vi "MotionProfileUpdater.vi"(11 "Main MP Controller In":T1={"DeviceStatus"={"status"=FALSE, "code"=0, "source"=""}, "Type"=enum."PWM", "PWM"={"PWM Channel"=enum."Invalid", "DeadBand"={"Name"="", "maxPositivePwm"=0, "minPositivePwm"=0, "centerPwm"=0, "maxNegativePwm"=0, "minNegativePwm"=0, "angularRange"=0}}, "CAN"={"Device Number"=0, "SetOutput VI Ref"=variant(enum8{"Percent VBus", "Current", "Speed", "Position", "Voltage"} enum."Percent VBus"), "GetOutput VI Ref"=variant(refnum<k1> refnum), "Enable VI Ref"=variant(dbl 12.0), "Disable VI Ref"=variant(enum8{"Percent VBus", "Speed", "Position", "Slave", "Unchanged / Invalid", "Voltage Compensation", "Current", "Motion Profile"} enum."Percent VBus"), "Data"=variant}, "Invert"=FALSE, "DIO PWM"={"PWM \"Enable\" Channel"=enum."Invalid", "DIOChannel"=enum."Invalid", "PWM Rate"=0.0}}) -> ()   [LabVIEW 2017]
uses:
  <vilib>/Rock Robotics/WPI/MotorControl/WPI_MotorControlDeviceRef.ctl
  <vilib>/Rock Robotics/WPI/MotorControl/WPI_MotorControlType.ctl
  <vilib>/Rock Robotics/SystemInterfaces/DIO/FPGA_DIOPWMChannel.ctl
  <vilib>/Rock Robotics/WPI/PWM/WPI_PWMDeadband.ctl
  <vilib>/Rock Robotics/SystemInterfaces/DIO/FPGA_DIOChannel.ctl
  TrajectoryPointCluster.ctl
  <vilib>/Rock Robotics/WPI/ThirdParty/Phoenix-LabVIEW/Motor Controller/Controls/CTRE_Phoenix_MotorControl_StatusFrameEnhanced.ctl
  <vilib>/Rock Robotics/WPI/ThirdParty/Phoenix-LabVIEW/Motor Controller/Controls/CTRE_Phoenix_MotorControl_ControlFrameEnhanced.ctl
  <vilib>/Rock Robotics/WPI/ThirdParty/Phoenix-LabVIEW/Motor Controller/Controls/CTRE_Phoenix_MotorControl_TrajectoryPointTimeDur.ctl
  MotionProfileController.vi
  Constants.vi
panel:
  out "Loop Rate (ms)":u32
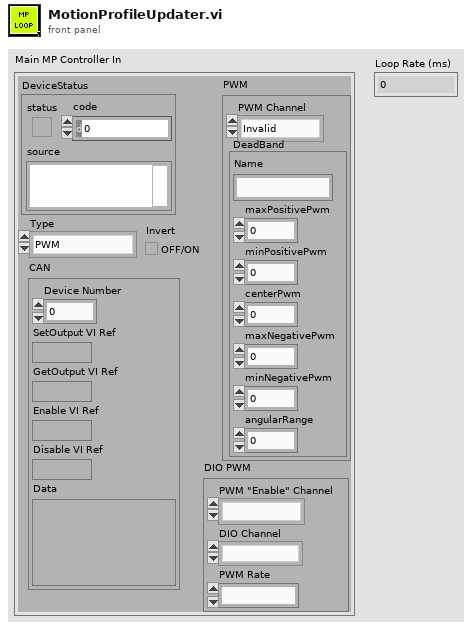
[diagram p1: front panel]
types:
  T1 = typedef "WPI_MotorControlDeviceRef.ctl" = cluster{"DeviceStatus":errorcluster, "Type":T2, "PWM":cluster{"PWM Channel":T3, "DeadBand":T4}, "CAN":cluster{"Device Number":u8, "SetOutput VI Ref":variant, "GetOutput VI Ref":variant, "Enable VI Ref":variant, "Disable VI Ref":variant, "Data":variant}, "Invert":bool, "DIO PWM":cluster{"PWM \"Enable\" Channel":T3, "DIOChannel":T5, "PWM Rate":dbl}}
  T2 = typedef "WPI_MotorControlType.ctl" = enum16{"PWM", "CAN", "DIO PWM"}
  T3 = typedef "FPGA_DIOPWMChannel.ctl" = enum8{"PWM 0", "PWM 1", "PWM 2", "PWM 3", "PWM 4", "PWM 5", "PWM 6", "PWM 7", "PWM 8", "PWM 9", "PWM MXP 0", "PWM MXP 1", "PWM MXP 2", "PWM MXP 3", "PWM MXP 4", "PWM MXP 5", "PWM MXP 6", "PWM MXP 7", "PWM MXP 8", "PWM MXP 9", "Invalid"}
  T4 = typedef "WPI_PWMDeadband.ctl" = cluster{"Name":string, "maxPositivePwm":i32, "minPositivePwm":i32, "centerPwm":i32, "maxNegativePwm":i32, "minNegativePwm":i32, "angularRange":u16}
  T5 = typedef "FPGA_DIOChannel.ctl" = enum8{"DIO 0", "DIO 1", "DIO 2", "DIO 3", "DIO 4", "DIO 5", "DIO 6", "DIO 7", "DIO 8", "DIO 9", "DIO MXP 0", "DIO MXP 1", "DIO MXP 2", "DIO MXP 3", "DIO MXP 4", "DIO MXP 5", "DIO MXP 6", "DIO MXP 7", "DIO MXP 8", "DIO MXP 9", "DIO MXP 10", "DIO MXP 11", "DIO MXP 12", "DIO MXP 13", "DIO MXP 14", "DIO MXP 15", "SPI Port CS1", "SPI Port CS2", "SPI Port CS3", "SPI Port MISO", "SPI Port MOSI", "Invalid"}
  T6 = typedef "CTRE_Phoenix_MotorControl_ControlFrameEnhanced.ctl" = u32
  T7 = typedef "CTRE_Phoenix_MotorControl_StatusFrameEnhanced.ctl" = u16
  T8 = typedef "TrajectoryPointCluster.ctl" = cluster{"Position":dbl, "Velocity":dbl, "Heading":dbl, "Time":dbl}
  T9 = cluster{"Top Buffer Remaining":i32, "Top Buffer Count":i32, "Bottom Buffer Count":i32, "Has Underrun?":bool, "Is Underrun?":bool, "Active Point Valid?":bool, "Is Last?":bool, "Profile Slot Select 0":i32, "Output Enable":i32, "Time Duration (ms)":i32, "Profile Slot Select 1":i32}
  T10 = typedef "CTRE_Phoenix_MotorControl_TrajectoryPointTimeDur.ctl" = i32
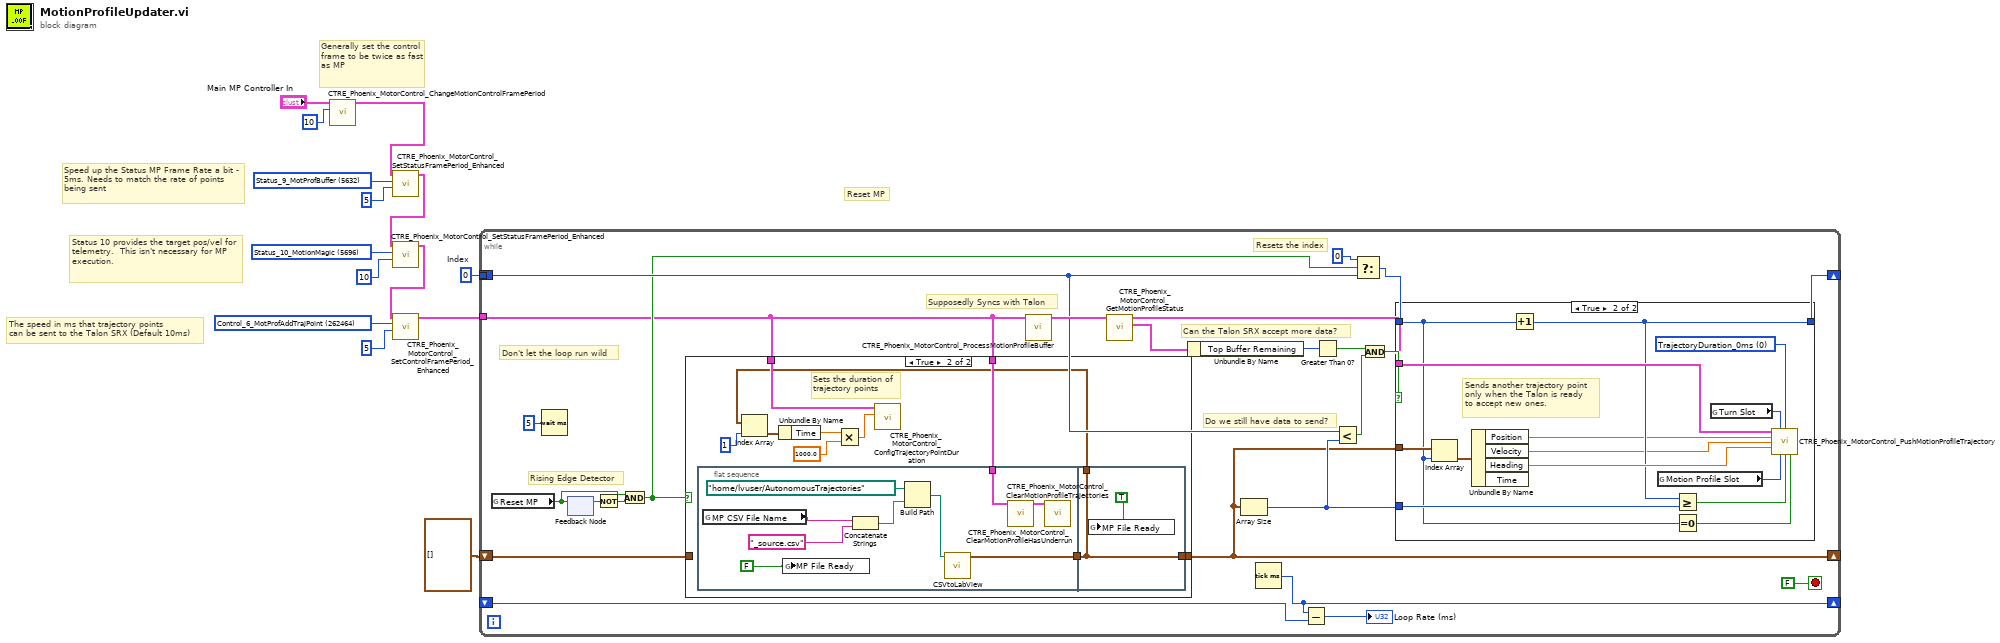
[diagram p0: block diagram]
diagram:
  w5 = T6 262464 items=["Control_3_General"=262272, "Control_4_Advanced"=262336, "Control_5_FeedbackOutputOverride"=262400, "Control_6_MotProfAddTrajPoint"=262464] ("Control Frame")
  w9 = T7 5696 items=["Status_1_General"=5120, "Status_2_Feedback0"=5184, "Status_3_Quadrature"=5248, "Status_4_AinTempVbat"=5312, "Status_6_Misc"=5440, "Status_7_CommStatus"=5504, "Status_8_PulseWidth"=5568, "Status_9_MotProfBuffer"=5632, "Status_10_MotionMagic"=5696, "Status_11_UartGadgeteer"=5760, "Status_12_Feedback1"=5824, "Status_13_Base_PIDF0"=5888, "Status_14_Turn_PIDF1"=5952, "Status_15_FirmwareApiStatus"=6016] ("Status Frame")
  w11 = T7 5632 items=["Status_1_General"=5120, "Status_2_Feedback0"=5184, "Status_3_Quadrature"=5248, "Status_4_AinTempVbat"=5312, "Status_6_Misc"=5440, "Status_7_CommStatus"=5504, "Status_8_PulseWidth"=5568, "Status_9_MotProfBuffer"=5632, "Status_10_MotionMagic"=5696, "Status_11_UartGadgeteer"=5760, "Status_12_Feedback1"=5824, "Status_13_Base_PIDF0"=5888, "Status_14_Turn_PIDF1"=5952, "Status_15_FirmwareApiStatus"=6016] ("Status Frame")
  w14 = 0  # Index
  # "Reset MP"
  # "The speed in ms that trajectory points\ncan be sent to the Talon SRX (Default 10ms)"
  # "Generally set the control frame to be twice as fast as MP"
  # "Status 10 provides the target pos/vel for telemetry.  This isn't necessary for MP execution."
  # "Speed up the Status MP Frame Rate a bit - 5ms. Needs to match the rate of points\nbeing sent"
  n1 = call <vilib>:"CTRE_Phoenix_MotorControl_ChangeMotionControlFramePeriod.vi"("periodMs"=10, "PhoenixMotorControlDevRef"="Main MP Controller In") -> ("PhoenixMotorControlDevRef"=w1:T1)  [unwired: 8 in, 1 out]
  n2 = call <vilib>:"CTRE_Phoenix_MotorControl_SetStatusFramePeriod_Enhanced.vi"("periodMs"=5, "Status Frame"=w11, "PhoenixMotorControlDevRef"=w1) -> ("PhoenixMotorControlDevRef"=w7:T1)  [unwired: 7 in, 1 out]
  n3 = call <vilib>:"CTRE_Phoenix_MotorControl_SetStatusFramePeriod_Enhanced.vi"("periodMs"=10, "Status Frame"=w9, "PhoenixMotorControlDevRef"=w7) -> ("PhoenixMotorControlDevRef"=w4:T1)  [unwired: 7 in, 1 out]
  n4 = call <vilib>:"CTRE_Phoenix_MotorControl_SetControlFramePeriod_Enhanced.vi"("periodMs"=5, "Control Frame"=w5, "MotorControl Device Ref"=w4) -> ("PhoenixMotorControlDevRef"=w12:T1)  [unwired: 7 in, 1 out]
  n5 = while {
    shift-right: [w36] -> _
    shift-left: w14 -> [w31]
    tunnel: w14 -> [_]
    tunnel: w12 -> [w15]
    shift-right: [w21] -> _
    shift-left: T8[] [] ("Trajectory Point Array") -> [w16]
    shift-right: [w20] -> _
    shift-left: _ -> [w19]
    stop <- FALSE stop-if-true
    # "Supposedly Syncs with Talon"
    # "Resets the index"
    # "Don't let the loop run wild"
    # "Do we still have data to send?"
    # "Can the Talon SRX accept more data?"
    # "Rising Edge Detector"
    n6 = global read "MotionProfileController.vi" "Reset MP"() -> (w17:bool)
    n7 = Wait (ms)(milliseconds to wait=u32 5) -> ()  [unwired: 1 out]
    n8 = feedback-in #1(w17) -> ()
    n9 = feedback #1() -> (w24:bool)  [unwired: 1 in]
    n10 = Not(x=w24) -> (.not. x?=w23:bool)
    n11 = And(x=w17, y=w23) -> (x .and. y?=w22:bool)
    n12 = case shown="True" w22 {
      tunnel: w15 -> [_ w49]
      tunnel: [w39 w48] -> w21
      tunnel: w16 -> [w39 _]
      tunnel: w15 -> [_ w43]
      frame False {
      }
      frame True {
        # "Sets the duration of\ntrajectory points"
        n13 = flat-sequence {
          tunnel: w49 -> [w53]
          tunnel: [w52] -> w47
          tunnel: [w59] -> w48
          tunnel: w47 -> [w59]
          tunnel: [w59] -> w42
          frame #0 {
            n14 = global read "MotionProfileController.vi" "MP CSV File Name"() -> (w50:string)
            n15 = global write "MotionProfileController.vi" "MP File Ready"(FALSE ("MP Ready")) -> ()
            n16 = Concatenate Strings(w50, "_source.csv") -> (w56:string)
            n17 = Build Path(base path=path "/home/lvuser/AutonomousTrajectories", name or relative path=w56) -> (appended path=w55:path)
            n18 = call "CSVtoLabView.vi"("file path (dialog if empty)"=w55) -> ("Trajectory Point Array"=w52:T8[])  [unwired: 10 in]
            n19 = call <vilib>:"CTRE_Phoenix_MotorControl_ClearMotionProfileTrajectories.vi"("PhoenixMotorControlDevRef"=w53) -> ("PhoenixMotorControlDevRef"=w54:T1)  [unwired: 13 in, 1 out]
            n20 = call <vilib>:"CTRE_Phoenix_MotorControl_ClearMotionProfileHasUnderrun.vi"("PhoenixMotorControlDevRef"=w54) -> ()  [unwired: 9 in, 2 out]
          }
          frame #1 {
            n21 = global write "MotionProfileController.vi" "MP File Ready"(TRUE ("MP Ready")) -> ()
          }
        }
        n22 = Index Array(array=w42, index=1) -> (element=w41:T8)
        n23 = Unbundle By Name(w41) -> ("Time"=w40:dbl)
        n24 = Multiply(x=w40, y=1000.0) -> (x*y=w46:dbl)
        n25 = call <vilib>:"CTRE_Phoenix_MotorControl_ConfigTrajectoryPointDuration.vi"("durationMs"=w46, "PhoenixMotorControlDevRef"=w43) -> ()  [unwired: 8 in, 2 out]
      }
    }
    n26 = call <vilib>:"CTRE_Phoenix_MotorControl_ProcessMotionProfileBuffer.vi"("PhoenixMotorControlDevRef"=w15) -> ("PhoenixMotorControlDevRef"=w32:T1)  [unwired: 13 in, 1 out]
    n27 = call <vilib>:"CTRE_Phoenix_MotorControl_GetMotionProfileStatus.vi"("PhoenixMotorControlDevRef"=w32) -> ("Motion Profile Status"=w33:T9, "PhoenixMotorControlDevRef"=w25:T1)  [unwired: 8 in, 1 out]
    n28 = Unbundle By Name(w33) -> ("Top Buffer Remaining"=w29:i32)
    n29 = Array Size(array=w21) -> (size(s)=w30:i32)
    n30 = Tick Count (ms)() -> (millisecond timer value=w20:u32)
    n31 = Subtract(x=w20, y=w19) -> (x-y=→"Loop Rate (ms)":u32)
    n32 = Greater Than 0?(x=w29) -> (x > 0?=w28:bool)
    n33 = Less?(x=w31, y=w30) -> (x < y?=w38:bool)
    n34 = Select(t=0, s=w22, f=w31) -> (s? t:f=w27:i32)
    n35 = And(x=w28, y=w38) -> (x .and. y?=w37:bool)
    n36 = case shown="True" w37 {
      tunnel: w21 -> [_ w75]
      tunnel: w25 -> [_ w72]
      tunnel: w30 -> [_ w70]
      tunnel: [w61 w67] -> w36
      tunnel: w27 -> [w61 w64]
      frame False {
      }
      frame True {
        w68 = T10 0 items=["TrajectoryDuration_0ms"=0, "TrajectoryDuration_5ms"=5, "TrajectoryDuration_10ms"=10, "TrajectoryDuration_20ms"=20, "TrajectoryDuration_30ms"=30, "TrajectoryDuration_40ms"=40, "TrajectoryDuration_50ms"=50, "TrajectoryDuration_100ms"=100] ("durationMs")
        # "Sends another trajectory point\nonly when the Talon is ready\nto accept new ones."
        n37 = Index Array(array=w75, index=w64) -> (element=w74:T8)
        n38 = Unbundle By Name(w74) -> ("Position"=w66:dbl, "Velocity"=w65:dbl, "Heading"=w73:dbl)  [unwired: 1 out]
        n39 = Increment(x=w64) -> (x+1=w67:i32)
        n40 = global read "Constants.vi" "Motion Profile Slot"() -> (w62:i32)
        n41 = Greater Or Equal?(x=w67, y=w70) -> (x >= y?=w69:bool)
        n42 = Equal To 0?(x=w64) -> (x = 0?=w71:bool)
        n43 = global read "Constants.vi" "Turn Slot"() -> (w63:i32)
        n44 = call <vilib>:"CTRE_Phoenix_MotorControl_PushMotionProfileTrajectory.vi"("PhoenixMotorControlDevRef"=w72, "profileSlotSelect1"=w63, "durationMs"=w68, "position"=w66, "velocity"=w65, "auxiliaryPos"=w73, "profileSlotSelect0"=w62, "isLastPoint?"=w69, "Zero Position?"=w71) -> ()  [unwired: 5 in, 2 out]
      }
    }
  }
